vi "Get Fit Plot Name.vi"(5 "Fit Algorithm":T1, 7 "Weighted Histogram Fit":bool, 9 "Fit Model":string, 10 "Plot Name":string, 11 "Fit Method":T2 items=["Least Square", "Least Absolute Residual", "Bisquare"]) -> (2 "Fit Plot Name":string)   [LabVIEW 2019]
uses:
  <vilib>/Analysis/6fits.llb/Curve Fitting Criteria.ctl
  Fit Algorithm.ctl
  <vilib>/Analysis/NI_AALPro.lvlib
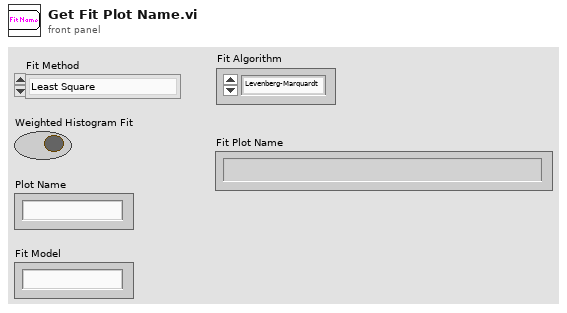
[diagram p1: front panel]
types:
  T1 = typedef "Fit Algorithm.ctl" = enum16{"Levenberg-Marquardt", "Trust-Region Dogleg"}
  T2 = typedef "NI_AALPro.lvlib/Curve Fitting Criteria.ctl" = u16
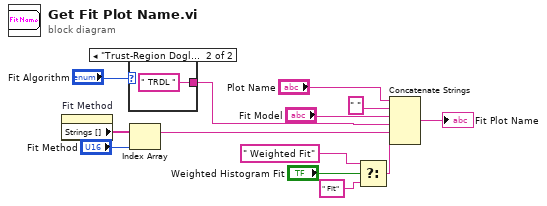
[diagram p0: block diagram]
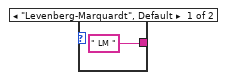
[diagram p2: hidden frame]
diagram:
  n1 = property on="Fit Method" class="Ring (strict)"() -> ("Strings []"=w6:string[])  [unwired: 2 in, 2 out]
  n2 = case shown="\"Trust-Region Dogleg\"" "Fit Algorithm" {
    tunnel: [" LM " ("string") " TRDL " ("string")] -> w1
    frame "Levenberg-Marquardt", Default {
    }
    frame "Trust-Region Dogleg" {
    }
  }
  n3 = Index Array(array=w6, index="Fit Method") -> (element=w4:string)
  n4 = Select(t=" Weighted Fit" ("string"), s="Weighted Histogram Fit", f=" Fit" ("string")) -> (s? t:f=w9:string)
  n5 = Concatenate Strings("Plot Name", " " ("string"), "Fit Model", w1, w4, w9) -> (→"Fit Plot Name":string)
